vi "Set Multi.vi"(0 "Display State In":T2, 5 "Value In":T1, 7 "First?":bool, 9 "Container State":T3, 11 "error in (no error)":errorcluster) -> (4 "Display State Out":T2, 15 "error out":errorcluster)   [LabVIEW 2015, in "Vowel.xctl"]
uses:
  Vowel.xctl
  <vilib>/_xctls/Container State.ctl
  State.ctl
  Vowel.Properties.ctl
  Utility VIs/Controls/KCheckbox/KCheckbox.xctl
  <vilib>/_xctls/XControlSupport.lvlib
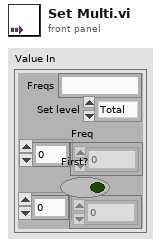
[diagram p1: front panel]
types:
  T1 = typedef "Vowel.xctl/Vowel.Properties.ctl" = cluster{"Freqs":string, "Set level":enum16{"Total", "Per component"}, "Freq":dbl[], "weights":dbl[]}
  T2 = typedef "Vowel.xctl/State.ctl" = cluster{"enable menu":bool, "ctls":cluster{"Freq":refnum<vi>, "Phase":refnum<vi>}}
  T3 = typedef "XControlSupport.lvlib/Container State.ctl" = cluster{"Indicator?":bool, "Run Mode?":bool, " Refnum":refnum<vi>}
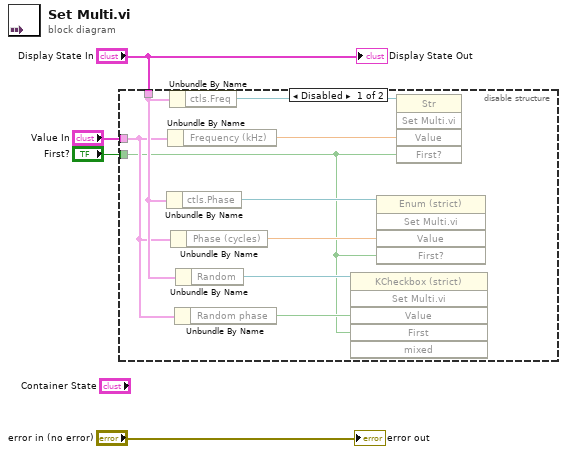
[diagram p0: block diagram]
diagram:
  n1 = disable-structure shown="Disabled" {
    disable-tunnel: "Display State In" -> [w10 _]
    disable-tunnel: "Value In" -> [w8 _]
    disable-tunnel: "First?" -> [w6 _]
    frame Disabled {
      n2 = Unbundle By Name(w10) -> ("ctls.Phase"=w12:refnum<vi>)
      n3 = Unbundle By Name(w8) -> ("Frequency (kHz)"=w5:dbl)
      n4 = Unbundle By Name(w10) -> ("ctls.Freq"=w13:refnum<vi>)
      n5 = Unbundle By Name(w8) -> ("Phase (cycles)"=w11:dbl)
      n6 = Unbundle By Name(w8) -> ("Random phase"=w7:bool)
      n7 = Unbundle By Name(w10) -> ("Random"=w9:refnum<vi>)
      n8 = invoke class="KCheckbox (strict)" method="Set Multi.vi"(reference=w9, "Value"=w7, "First"=w6) -> ()  [unwired: 3 in, 6 out]
      n9 = invoke class="Enum (strict)" method="Set Multi.vi"(reference=w12, "Value"=w11, "First?"=w6) -> ()  [unwired: 2 in, 5 out]
      n10 = invoke class="Str" method="Set Multi.vi"(reference=w13, "Value"=w5, "First?"=w6) -> ()  [unwired: 2 in, 5 out]
    }
    frame Enabled {
    }
  }
  "Display State Out" <- "Display State In"
  "error out" <- "error in (no error)"
